vi "Octave Range to Band Number.vi"(1 "frequency range":T1={"low band"=enum."1000 Hz", "high band"=enum."1000 Hz"}) -> (0 "band number":cluster{"low band":i32, "high band":i32})   [LabVIEW 2017]
doc: "Converts the selected octave frequency range to the corresponding band number.\nThe band number is based on the low and high bands specified in the frequency range cluster. A value of 0 corresponds to the reference frequency of the audio-frequency range, 1 kHz. Each successive value corresponds to the next octave band. Positive values cover the range above 1 kHz, and negative values cover the range below 1 kHz.\nThe frequency range cluster uses a pre-defined list of frequencies from 16 Hz to 16 kHz, in octave steps. If you need to use any other specific frequency outside of this frequency range, use the Frequency Range to Band Number VI instead."
uses:
  <vilib>/addons/Sound and Vibration/svt_Octave/SoundVib_Octave_2014 standard.lvlib
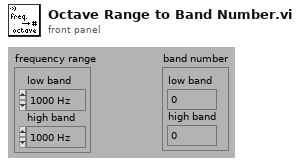
[diagram p1: front panel]
types:
  T1 = cluster{"low band":enum16{"16 Hz", "31.5 Hz", "63 Hz", "125 Hz", "250 Hz", "500 Hz", "1000 Hz", "2000 Hz", "4000 Hz", "8000 Hz", "16000 Hz"}, "high band":enum16{"16 Hz", "31.5 Hz", "63 Hz", "125 Hz", "250 Hz", "500 Hz", "1000 Hz", "2000 Hz", "4000 Hz", "8000 Hz", "16000 Hz"}}
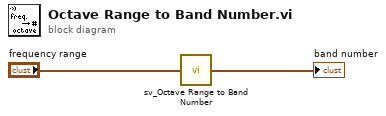
[diagram p0: block diagram]
diagram:
  n1 = call <vilib>:"sv_Octave Range to Band Number.vi"("frequency range"="frequency range") -> ("band number"=→"band number":cluster{"low band":i32, "high band":i32})
